vi "To Serial Form.vi"(6 "Serial Version":T1, 10 "Serializer in":refnum<class "Serializer.lvclass">, 11 "BrowerComposite in":refnum<class "BrowerComposite.lvclass">) -> (0 "error out":errorcluster, 2 "Serializer out":refnum<class "Serializer.lvclass">, 3 "BrowerComposite out":refnum<class "BrowerComposite.lvclass">)   [LabVIEW 2015, in "BrowerComposite.lvclass"]
uses:
  BrowerComposite.lvclass
  <vilib>/NI/AQ Character Lineator/Serializer/Serializer.lvclass
  <vilib>/NI/AQ Character Lineator/Serialization Common/Serial Version.ctl
  <vilib>/NI/AQ Character Lineator/Serializable/Insert Serializable Array.vi
  <vilib>/NI/AQ Character Lineator/Serializable/Insert String Array.vi
  <vilib>/NI/AQ Character Lineator/Serializable/Insert Serializable.vi
  <vilib>/NI/AQ Character Lineator/Serializer/Insert String Array.vi
  <vilib>/NI/AQ Character Lineator/Serializer/Insert Serializable Array.vi
  <vilib>/NI/AQ Character Lineator/Serializer/Read Include Default Values.vi
  <vilib>/NI/AQ Character Lineator/Serializer/Insert Serializable.vi
  BrowerComponent/BrowerComponent.lvclass
  <vilib>/NI/AQ Character Lineator/Serializable/Serializable.lvclass
  <vilib>/NI/AQ Character Lineator/Serialization Common/Serialization Common.lvlib
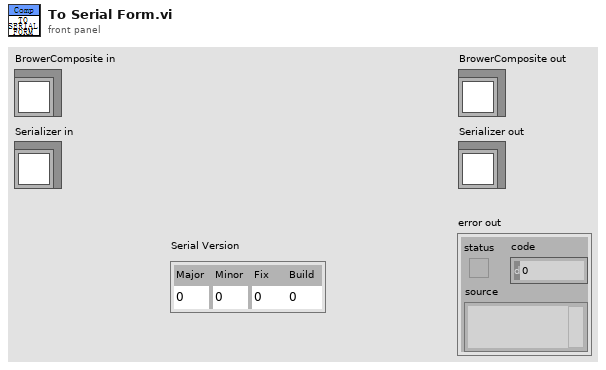
[diagram p1: front panel]
types:
  T1 = typedef "Serialization Common.lvlib/Serial Version.ctl" = cluster{"Major":u16, "Minor":u16, "Fix":u16, "Build":u16}
  T2 = typedef "BrowerComposite.lvclass/ObjectAttributes.ctl" = cluster{"BrowerComponents":refnum<class "BrowerComponent.lvclass">[], "BrowerComponentIDs":string[], "Iterator":refnum<class "Iterator.lvclass">}
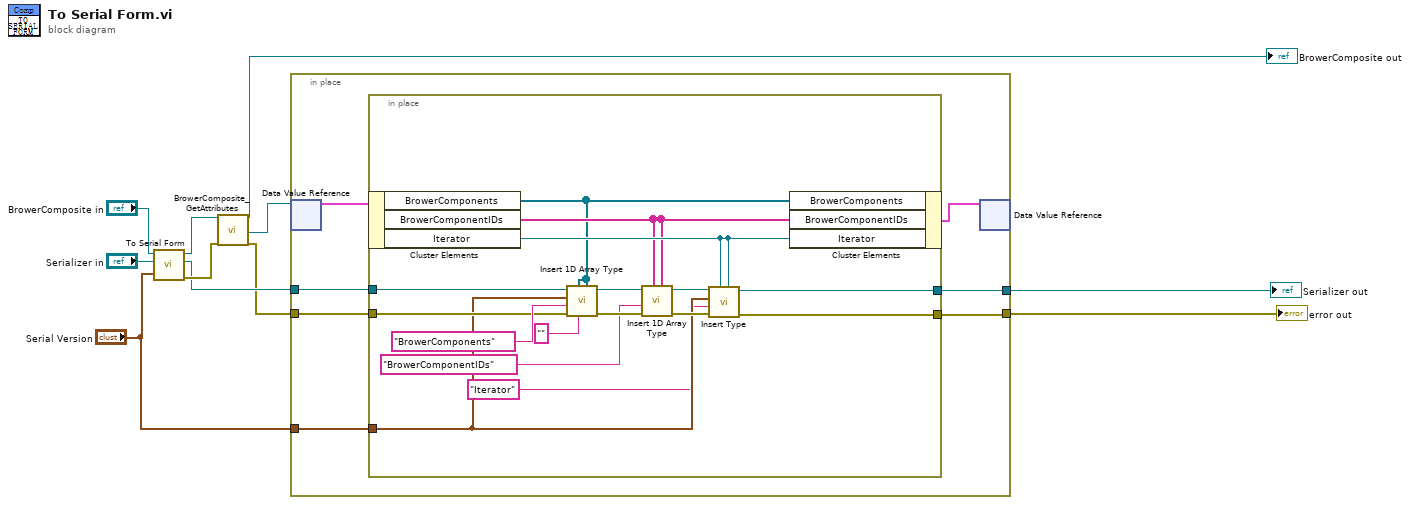
[diagram p0: block diagram]
diagram:
  n1 = call-parent "To Serial Form.vi"("Serial Version"="Serial Version", "Serializer in"="Serializer in", "BrowerComponent in"="BrowerComposite in") -> ("error out"=w8:errorcluster, "Serializer out"=w6:refnum<class "Serializer.lvclass">, "BrowerComponent out"=w9:refnum<class "BrowerComposite.lvclass">)  [unwired: 6 in]
  n2 = call "BrowerComposite_GetAttributes.vi"("reference in"=w9, "error in (no error)"=w8) -> ("reference out"=→"BrowerComposite out":refnum<class "BrowerComposite.lvclass">, "DataRef"=w7:refnum<data-value>, "error out"=w4:errorcluster)  [unwired: 14 in, 1 out]
  n3 = in-place {
    in-place-border: w6 -> [w17]
    in-place-border: "Serial Version" -> [w16]
    in-place-border: w4 -> [w15]
    in-place-border: [w13] -> w2
    in-place-border: [w12] -> w1
    n4 = in-place-dvr #1(w7) -> (w18:T2)  [unwired: 1 out]
    n5 = in-place {
      in-place-border: w17 -> [w34]
      in-place-border: w16 -> [w25]
      in-place-border: w15 -> [w29]
      in-place-border: [w20] -> w13
      in-place-border: [w19] -> w12
      n6 = in-place-cluster #2(w18) -> ("BrowerComponents"=w21:refnum<class "BrowerComponent.lvclass">[], "BrowerComponentIDs"=w22:string[], "Iterator"=w23:refnum<class "Iterator.lvclass">)
      n7 = call-poly <vilib>:"Insert 1D Array Type.vi"("Serializables"=w21, "Default Class Qualified Name"="", "Default Value"=w21, "error in (no error)"=w29, "Name"="BrowerComponents", "Serial Version"=w25, "Serializer in"=w34) -> ("error out"=w30:errorcluster, "Serializer out"=w31:refnum<class "Serializer.lvclass">)  [unwired: 3 in]
      n8 = call-poly <vilib>:"Insert 1D Array Type.vi"("Strings"=w22, "Default Value"=w22, "error in (no error)"=w30, "Name"="BrowerComponentIDs", "Serializer in"=w31) -> ("error out"=w26:errorcluster, "Serializer out"=w27:refnum<class "Serializer.lvclass">)  [unwired: 5 in]
      n9 = call-poly <vilib>:"Insert Type.vi"("Serializable"=w23, "Default Value"=w23, "error in (no error)"=w26, "Name"="Iterator", "Serial Version"=w25, "Serializer in"=w27) -> ("error out"=w19:errorcluster, "Serializer out"=w20:refnum<class "Serializer.lvclass">)  [unwired: 4 in]
      n10 = in-place-cluster #2("BrowerComponents"=w21, "BrowerComponentIDs"=w22, "Iterator"=w23) -> (w14:T2)
    }
    n11 = in-place-dvr #1(w14) -> ()  [unwired: 2 out]
  }
  "error out" <- w1
  "Serializer out" <- w2
